vi "Read Channel names.vi"(8 "error in (no error)":errorcluster, 11 "Find Peaks Result in":refnum<class "Find Peaks Result.lvclass">) -> (0 "error out":errorcluster, 2 "Channel names":string[](array[string]), 3 "Find Peaks Result out":refnum<class "Find Peaks Result.lvclass">)   [LabVIEW 2015, in "Find Peaks Result.lvclass"]
uses:
  Find Peaks Result.lvclass
  Find Peaks Result.lvclass/Find Peaks Result.ctl
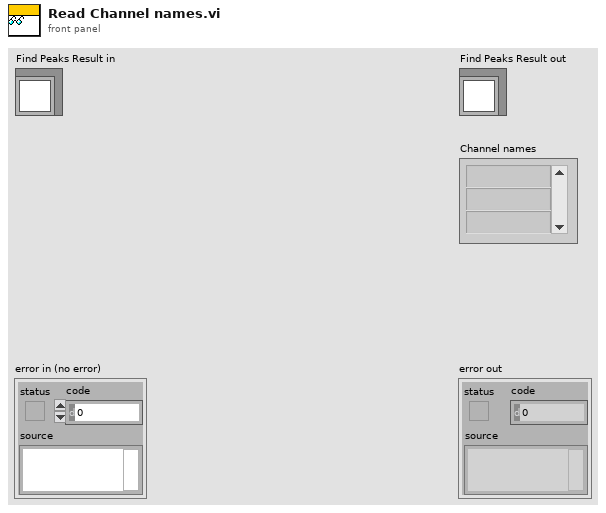
[diagram p1: front panel]
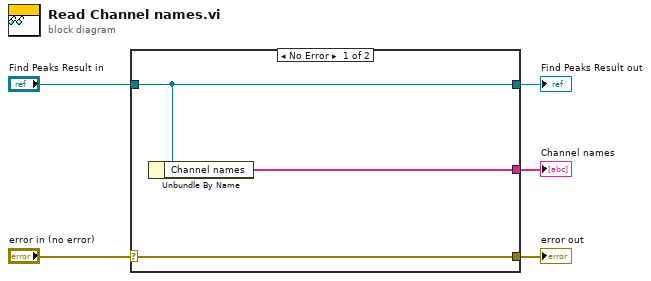
[diagram p0: block diagram]
diagram:
  n1 = case shown="No Error" "error in (no error)" {
    selector: "error in (no error)" -> [w8 w9]
    tunnel: [w8 w9] -> w4
    tunnel: [w7 w10] -> w2
    tunnel: "Find Peaks Result in" -> [w7 w10]
    tunnel: [w6 _] -> w1
    frame No Error {
      n2 = Unbundle By Name(w7) -> ("Channel names"=w6:string[])
    }
    frame Error {
    }
  }
  "error out" <- w4
  "Find Peaks Result out" <- w2
  "Channel names" <- w1
